vi "Ctor.vi"(8 "error in (no error)":errorcluster) -> (0 "error out":errorcluster, 3 "LV-Term App out":refnum<class "LV-Term App.lvclass">)   [LabVIEW 2020, in "LV-Term.lvlib" / "LV-Term App.lvclass"]
uses:
  LV-Term App.lvclass
  LV-Term App.lvclass/LV-Term App.ctl
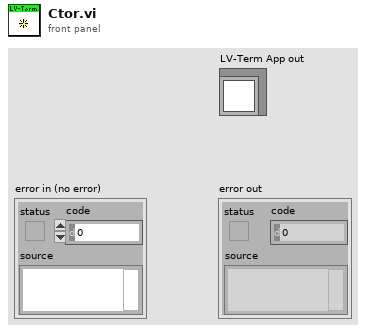
[diagram p1: front panel]
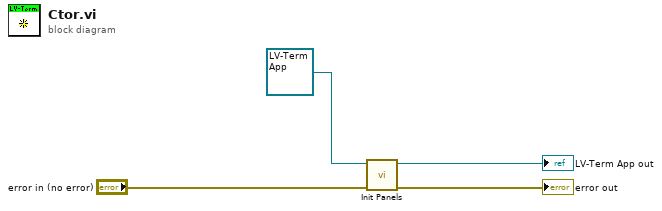
[diagram p0: block diagram]
diagram:
  n1 = call "Init Panels.vi"("error in (no error)"="error in (no error)", "LV-Term App in"=refnum<class "LV-Term App.lvclass"> refnum) -> ("error out"=→"error out":errorcluster, "LV-Term App out"=→"LV-Term App out":refnum<class "LV-Term App.lvclass">)  [unwired: 8 in]
